vi "BLAS3 Utility(DBL).vi"(0 "A":T2, 1 "B/X":T2, 2 "C":T2, 3 "operation A":T1 items=["Direct", "Conjugated & Transposed", "Transposed"], 4 "operation B":T1 items=["Direct", "Conjugated & Transposed", "Transposed"], 6 "function":T3 items=["ddot/zdotu/zdotc", "daxpy/zaxpy", "dnrm2/dznrm2", "dasum/dzasum", "dcopy/zcopy", "dswap/zswap", "drotm", "drot/zdrot", "idamax/izamax", "idamin/izamin", "dgemv/zgemv", "dsymv/zhemv", "dtrmv/ztrmv", "dsyr/zher", "dsyr2/zher2", "dger/zgeru/zgerc", "dtrsv/ztrsv", "dgemm/zgemm", "dsymm/zsymm/zhemm", "dtrmm/ztrmm", "dsyrk/zsyrk/zherk", "dsyr2k/zsyr2k/zher2k", "dtrsm/ztrsm"]) -> (10 "lda":i32, 11 "m":i32, 12 "ldb/ldx":i32, 13 "n":i32, 14 "ldc":i32, 19 "k":i32)   [LabVIEW 2017, in "NI_AALBLAS.lvlib"]
uses:
  NI_AALBLAS.lvlib
  RealMatrix.ctl
  LV_Transpose.ctl
  Fucntion.ctl
  NI_Matrix.lvlib
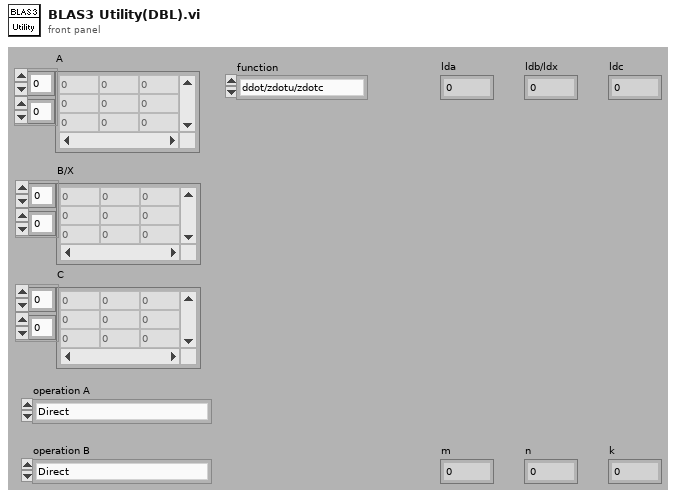
[diagram p1: front panel]
types:
  T1 = typedef "NI_AALBLAS.lvlib/LV_Transpose.ctl" = i32
  T2 = typedef "NI_Matrix.lvlib/RealMatrix.ctl" = dbl[][]
  T3 = typedef "NI_AALBLAS.lvlib/Fucntion.ctl" = u16
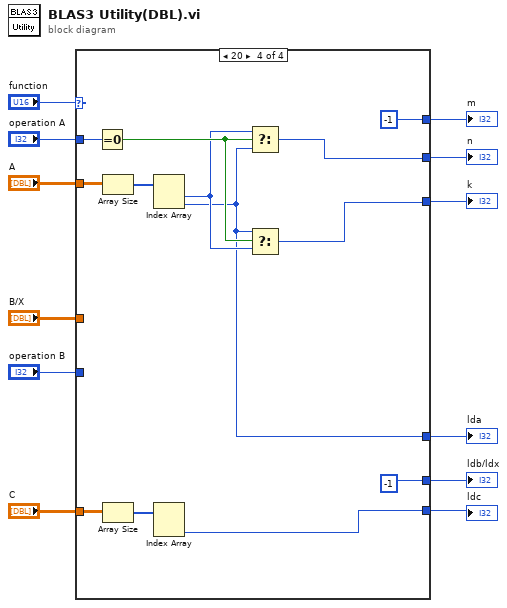
[diagram p0: block diagram]
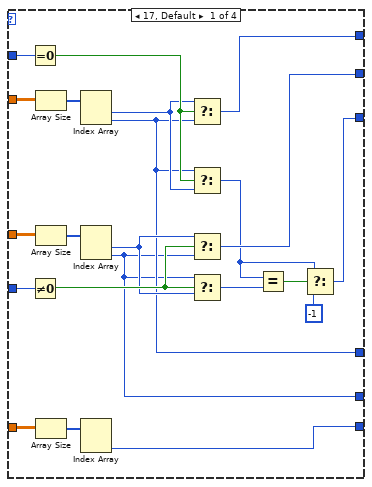
[diagram p2: hidden frame]
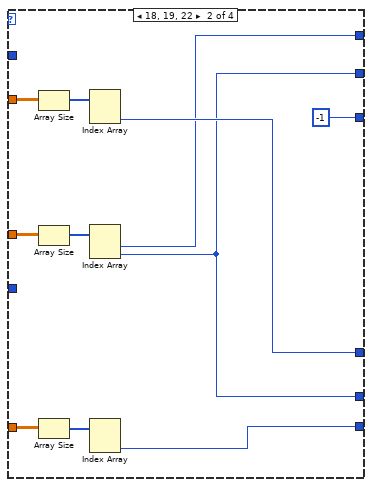
[diagram p3: hidden frame]
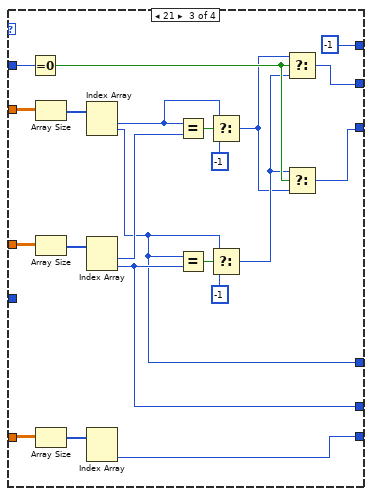
[diagram p4: hidden frame]
diagram:
  n1 = case shown="20" "function" {
    tunnel: "A" -> [w33 w37 w66 w79]
    tunnel: "operation A" -> [w31 _ w53 w80]
    tunnel: [w34 w36 w50 w71] -> w11
    tunnel: [w30 w42 -1 -1] -> w10
    tunnel: [w17 w45 w47 w69] -> w8
    tunnel: [w18 -1 w54 w75] -> w6
    tunnel: "B/X" -> [w29 w44 w63 _]
    tunnel: "operation B" -> [w27 _ _ _]
    tunnel: "C" -> [w15 w39 w51 w72]
    tunnel: [w16 w36 w49 -1] -> w2
    tunnel: [w13 w35 w46 w68] -> w1
    frame 17, Default {
      n2 = Equal To 0?(x=w31) -> (x = 0?=w26:bool)
      n3 = Not Equal To 0?(x=w27) -> (x != 0?=w24:bool)
      n4 = Array Size(array=w33) -> (size(s)=w32:i32[])
      n5 = Array Size(array=w29) -> (size(s)=w28:i32[])
      n6 = Array Size(array=w15) -> (size(s)=w14:i32[])
      n7 = Index Array(array=w32) -> (element #1=w25:i32, element #2=w17:i32)  [unwired: 2 in]
      n8 = Index Array(array=w28) -> (element #1=w23:i32, element #2=w16:i32)  [unwired: 2 in]
      n9 = Index Array(array=w14) -> (element #2=w13:i32)  [unwired: 2 in, 1 out]
      n10 = Select(t=w25, s=w26, f=w17) -> (s? t:f=w30:i32)
      n11 = Select(t=w17, s=w26, f=w25) -> (s? t:f=w20:i32)
      n12 = Select(t=w23, s=w24, f=w16) -> (s? t:f=w34:i32)
      n13 = Select(t=w16, s=w24, f=w23) -> (s? t:f=w22:i32)
      n14 = Equal?(x=w20, y=w22) -> (x = y?=w21:bool)
      n15 = Select(t=w20, s=w21, f=-1) -> (s? t:f=w18:i32)
    }
    frame 18, 19, 22 {
      n16 = Array Size(array=w37) -> (size(s)=w38:i32[])
      n17 = Array Size(array=w44) -> (size(s)=w43:i32[])
      n18 = Array Size(array=w39) -> (size(s)=w40:i32[])
      n19 = Index Array(array=w38) -> (element #2=w45:i32)  [unwired: 2 in, 1 out]
      n20 = Index Array(array=w43) -> (element #1=w42:i32, element #2=w36:i32)  [unwired: 2 in]
      n21 = Index Array(array=w40) -> (element #2=w35:i32)  [unwired: 2 in, 1 out]
    }
    frame 21 {
      n22 = Equal To 0?(x=w53) -> (x = 0?=w67:bool)
      n23 = Array Size(array=w66) -> (size(s)=w65:i32[])
      n24 = Array Size(array=w63) -> (size(s)=w64:i32[])
      n25 = Array Size(array=w51) -> (size(s)=w52:i32[])
      n26 = Index Array(array=w65) -> (element #1=w57:i32, element #2=w47:i32)  [unwired: 2 in]
      n27 = Index Array(array=w64) -> (element #1=w58:i32, element #2=w49:i32)  [unwired: 2 in]
      n28 = Index Array(array=w52) -> (element #2=w46:i32)  [unwired: 2 in, 1 out]
      n29 = Equal?(x=w57, y=w58) -> (x = y?=w62:bool)
      n30 = Equal?(x=w47, y=w49) -> (x = y?=w59:bool)
      n31 = Select(t=w57, s=w62, f=-1) -> (s? t:f=w55:i32)
      n32 = Select(t=w47, s=w59, f=-1) -> (s? t:f=w56:i32)
      n33 = Select(t=w55, s=w67, f=w56) -> (s? t:f=w50:i32)
      n34 = Select(t=w56, s=w67, f=w55) -> (s? t:f=w54:i32)
    }
    frame 20 {
      n35 = Equal To 0?(x=w80) -> (x = 0?=w77:bool)
      n36 = Array Size(array=w79) -> (size(s)=w78:i32[])
      n37 = Array Size(array=w72) -> (size(s)=w73:i32[])
      n38 = Index Array(array=w78) -> (element #1=w76:i32, element #2=w69:i32)  [unwired: 2 in]
      n39 = Index Array(array=w73) -> (element #2=w68:i32)  [unwired: 2 in, 1 out]
      n40 = Select(t=w76, s=w77, f=w69) -> (s? t:f=w71:i32)
      n41 = Select(t=w69, s=w77, f=w76) -> (s? t:f=w75:i32)
    }
  }
  "n" <- w11
  "m" <- w10
  "lda" <- w8
  "k" <- w6
  "ldb/ldx" <- w2
  "ldc" <- w1
